vi "Senser.vi"(8 "error in (no error)":errorcluster caption="错误输入（无错误）") -> (0 "error out":errorcluster caption="错误输出", 1 "x = y?":bool, 2 "子字符串":string)   [LabVIEW 2018]
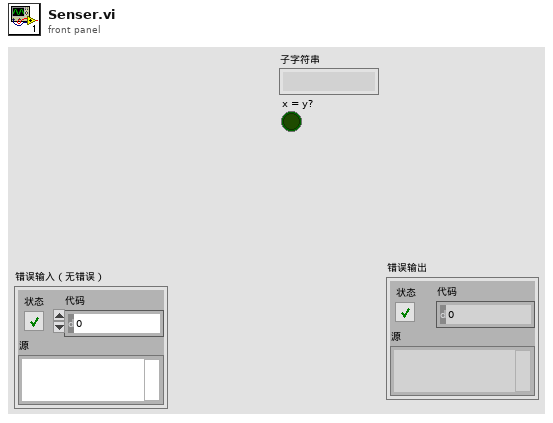
[diagram p1: front panel]
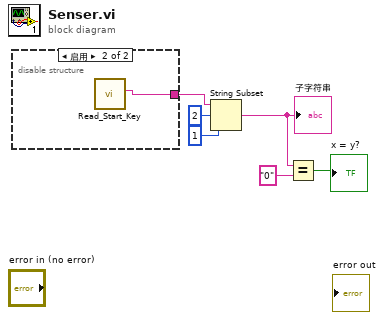
[diagram p0: block diagram]
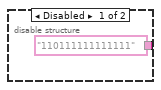
[diagram p2: hidden frame]
diagram:
  n1 = disable-structure shown="启用" {
    disable-tunnel: ["110111111111111" w8] -> w4
    frame Disabled {
    }
    frame Enabled {
      n2 = call "Read_Start_Key.vi"() -> ("子字符串之后"=w8:string)  [unwired: 8 in, 3 out]
    }
  }
  n3 = String Subset(string=w4, offset (0)=2 ("偏移量(0)"), length (rest)=1 ("长度（剩余）")) -> (substring=w3:string)
  "子字符串" <- w3
  n4 = Equal?(x=w3, y="0") -> (x = y?=→"x = y?":bool)
